vi "Menu.Enable Item.vi"(8 "error in":errorcluster, 9 "Enable":bool, 10 "Tag":string, 11 "Menu Ref":refnum<k9>) -> (0 "error out":errorcluster, 3 "Menu Ref Out":refnum<k9>)   [LabVIEW 2024, in "EQMF.lvlib" / "Menu Utils.lvlib"]
uses:
  Menu Utils.lvlib
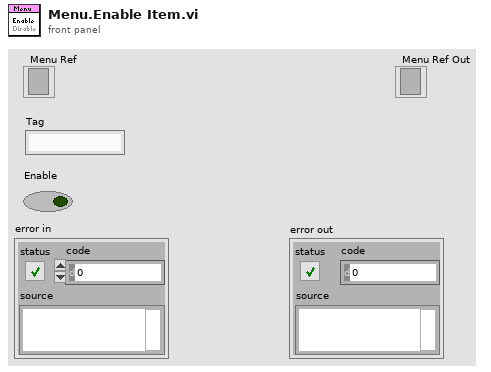
[diagram p1: front panel]
types:
  T1 = typedef "LVMenuShortCut.ctl" = cluster{"include Shift key?":bool, "include Ctrl key?":bool, "shortcut key":string}
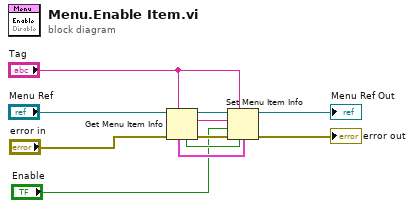
[diagram p0: block diagram]
diagram:
  n1 = Get Menu Item Info(7:"Tag", 8:"error in", 11:"Menu Ref") -> (0:w11:errorcluster, 2:w10:string, 3:w9:refnum<k9>, 4:w4:bool, 6:w8:T1)  [unwired: 2 out]
  n2 = Set Menu Item Info(4:w8, 6:w4, 7:"Tag", 8:w11, 9:"Enable", 10:w10, 11:w9) -> (0:→"error out":errorcluster, 3:→"Menu Ref Out":refnum<k9>)
